vi "graphs B (SubVI).vi"(10 "Cluster":T1) -> ()   [LabVIEW 2015]
uses:
  Load and Save Controls_LV2009.llb/RWC_Actions.ctl
  <vilib>/Utility/error.llb/DialogType.ctl
panel:
  out "1":dynamicdata(graph) caption="U, uV"
  out "2":dynamicdata(graph) caption="U, uV"
  out "3":dynamicdata(graph) caption="U, uV"
  out "4":dynamicdata(graph) caption="U, uV"
  out "5":dynamicdata(graph) caption="U, uV"
  out "6":dynamicdata(graph) caption="U, uV"
  out "7":dynamicdata(graph) caption="U, uV"
  out "8":dynamicdata(graph) caption="U, uV"
  in  "clrear graphs":bool
  in  "4 sc":bool=TRUE
  in  "5 sc":bool=TRUE
  in  "7 sc":bool=TRUE
  in  "1 sc":bool=TRUE
  in  "2 sc":bool=TRUE
  in  "3 sc":bool=TRUE
  in  "6 sc":bool=TRUE
  in  "8 sc":bool=TRUE
  in  "4":bool=TRUE
  in  "5":bool
  in  "7":bool
  in  "1":bool=TRUE
  in  "2":bool=TRUE
  in  "3":bool=TRUE
  in  "6":bool
  in  "8":bool
  in  "dec time":bool
  in  "inc time":bool
  in  "Добавить время":dbl(ring)=300.0 items=["1 мин."=60.0, "5 мин."=300.0, "20 мин."=1200.0]
  out "мин.":string="1"
  out "часы":string="0"
  # "№ канала"
  # ":"
  # "Вкл."
  # "Автошкала"
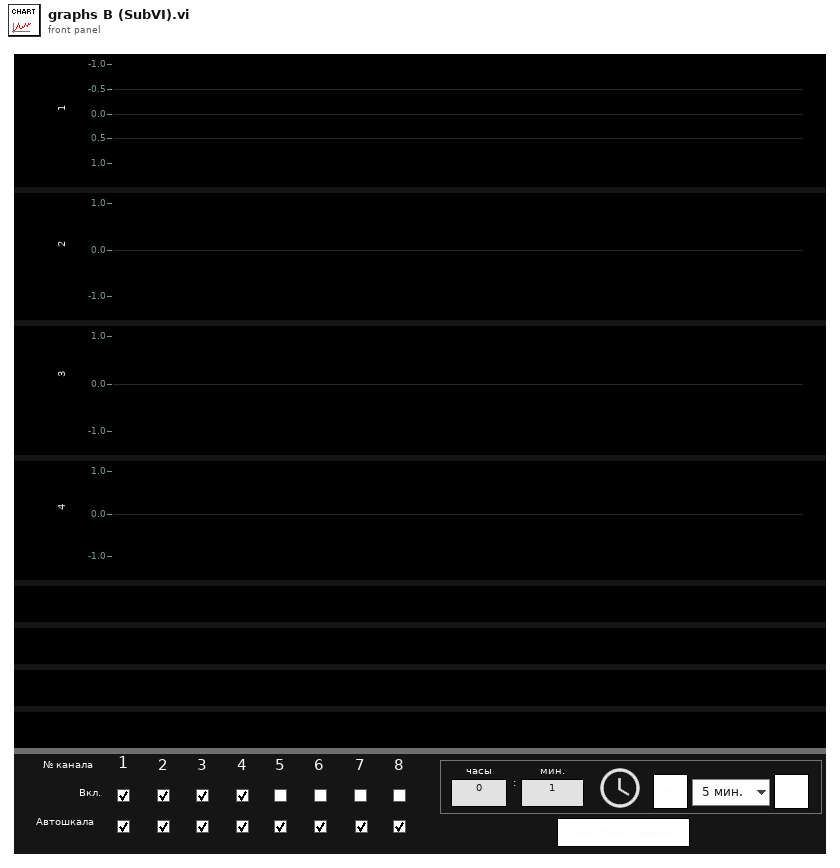
[diagram p1: front panel]
types:
  T1 = cluster{"1":dbl, "2":dbl, "3":dbl, "4":dbl, "5":dbl, "6":dbl, "7":dbl, "8":dbl}
  T2 = typedef "LVDateTimeRec.ctl" = cluster{"fractional second":dbl, "second":i32, "minute":i32, "hour":i32, "day of month":i32, "month":i32, "year":i32, "day of week":i32, "day of year":i32, "DST":i32}
  T3 = typedef "RWC_Actions.ctl" = enum16{"Read", "Write", "Read and Create"}
  T4 = typedef "DialogType.ctl" = u16
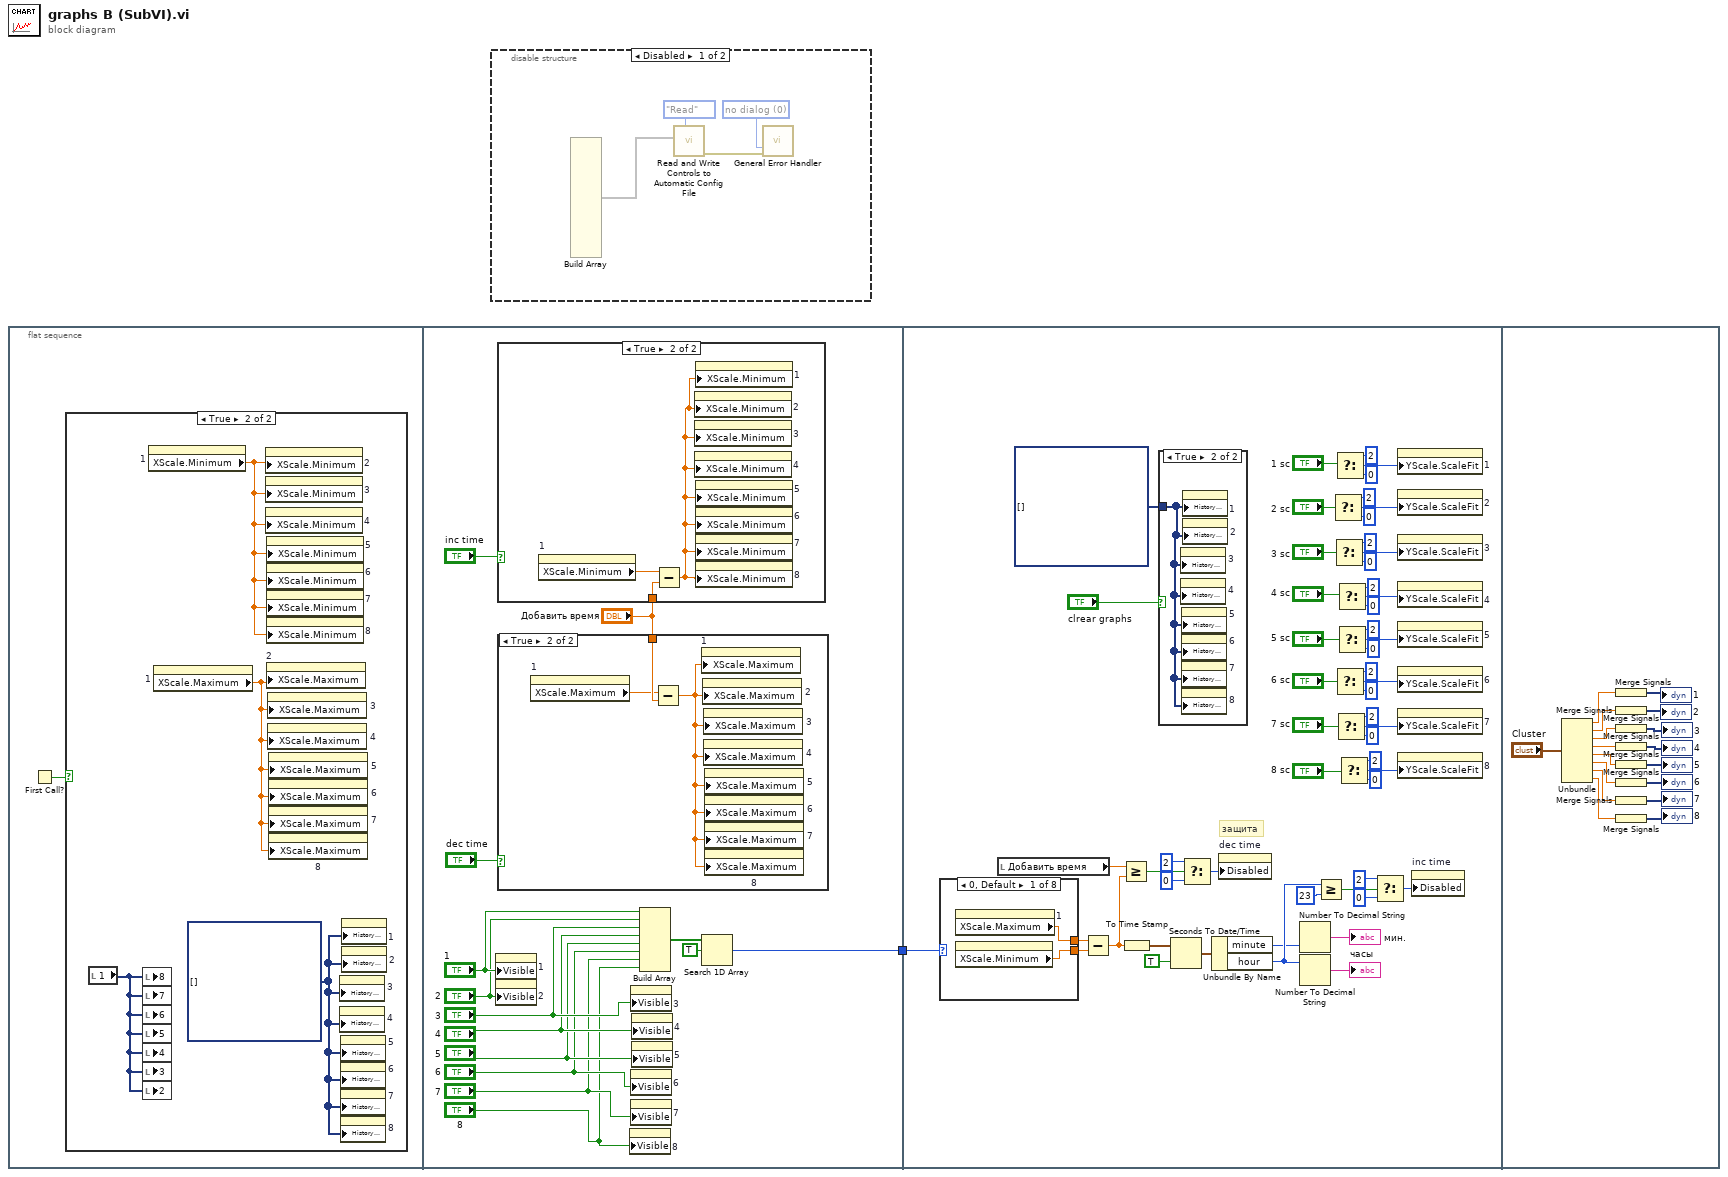
[diagram p0: block diagram]
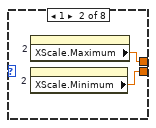
[diagram p7: hidden frame]
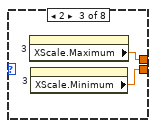
[diagram p8: hidden frame]
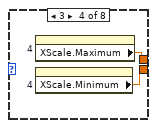
[diagram p9: hidden frame]
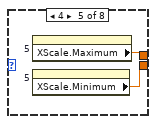
[diagram p10: hidden frame]
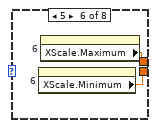
[diagram p11: hidden frame]
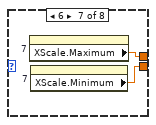
[diagram p12: hidden frame]
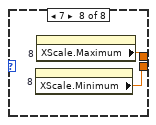
[diagram p13: hidden frame]
diagram:
  n1 = flat-sequence {
    tunnel: [w7] -> w1
    tunnel: w1 -> [w61]
    frame #0 {
      n2 = First Call?() -> (First Call?: T/F=w2:bool)
      n3 = case shown="True" w2 {
        frame False {
        }
        frame True {
          w6 = dynamicdata[] [] ("History Data")
          n4 = local read "1"() -> (w5:dynamicdata)
          n5 = local write "8"(w5) -> ()
          n6 = local write "7"(w5) -> ()
          n7 = local write "6"(w5) -> ()
          n8 = local write "5"(w5) -> ()
          n9 = local write "4"(w5) -> ()
          n10 = local write "3"(w5) -> ()
          n11 = local write "2"(w5) -> ()
          n12 = property on="1" class="WFChart (strict)"() -> ("XScale.Minimum"=w4:dbl)  [unwired: 2 in, 2 out]
          n13 = property on="1" class="WFChart (strict)"() -> ("XScale.Maximum"=w3:dbl)  [unwired: 2 in, 2 out]
          n14 = property on="2" class="WFChart (strict)"("XScale.Minimum"=w4) -> ()  [unwired: 2 in, 2 out]
          n15 = property on="3" class="WFChart (strict)"("XScale.Minimum"=w4) -> ()  [unwired: 2 in, 2 out]
          n16 = property on="4" class="WFChart (strict)"("XScale.Minimum"=w4) -> ()  [unwired: 2 in, 2 out]
          n17 = property on="5" class="WFChart (strict)"("XScale.Minimum"=w4) -> ()  [unwired: 2 in, 2 out]
          n18 = property on="6" class="WFChart (strict)"("XScale.Minimum"=w4) -> ()  [unwired: 2 in, 2 out]
          n19 = property on="7" class="WFChart (strict)"("XScale.Minimum"=w4) -> ()  [unwired: 2 in, 2 out]
          n20 = property on="8" class="WFChart (strict)"("XScale.Minimum"=w4) -> ()  [unwired: 2 in, 2 out]
          n21 = property on="2" class="WFChart (strict)"("XScale.Maximum"=w3) -> ()  [unwired: 2 in, 2 out]
          n22 = property on="3" class="WFChart (strict)"("XScale.Maximum"=w3) -> ()  [unwired: 2 in, 2 out]
          n23 = property on="4" class="WFChart (strict)"("XScale.Maximum"=w3) -> ()  [unwired: 2 in, 2 out]
          n24 = property on="5" class="WFChart (strict)"("XScale.Maximum"=w3) -> ()  [unwired: 2 in, 2 out]
          n25 = property on="6" class="WFChart (strict)"("XScale.Maximum"=w3) -> ()  [unwired: 2 in, 2 out]
          n26 = property on="7" class="WFChart (strict)"("XScale.Maximum"=w3) -> ()  [unwired: 2 in, 2 out]
          n27 = property on="8" class="WFChart (strict)"("XScale.Maximum"=w3) -> ()  [unwired: 2 in, 2 out]
          n28 = property on="3" class="WFChart (strict)"("History Data"=w6) -> ()  [unwired: 2 in, 2 out]
          n29 = property on="4" class="WFChart (strict)"("History Data"=w6) -> ()  [unwired: 2 in, 2 out]
          n30 = property on="5" class="WFChart (strict)"("History Data"=w6) -> ()  [unwired: 2 in, 2 out]
          n31 = property on="6" class="WFChart (strict)"("History Data"=w6) -> ()  [unwired: 2 in, 2 out]
          n32 = property on="7" class="WFChart (strict)"("History Data"=w6) -> ()  [unwired: 2 in, 2 out]
          n33 = property on="8" class="WFChart (strict)"("History Data"=w6) -> ()  [unwired: 2 in, 2 out]
          n34 = property on="1" class="WFChart (strict)"("History Data"=w6) -> ()  [unwired: 2 in, 2 out]
          n35 = property on="2" class="WFChart (strict)"("History Data"=w6) -> ()  [unwired: 2 in, 2 out]
        }
      }
    }
    frame #1 {
      n36 = property on="1" class="WFChart (strict)"("Visible"="1") -> ()  [unwired: 2 in, 2 out]
      n37 = property on="2" class="WFChart (strict)"("Visible"="2") -> ()  [unwired: 2 in, 2 out]
      n38 = case shown="True" "inc time" {
        tunnel: "Добавить время" -> [_ w26]
        frame False {
        }
        frame True {
          n39 = property on="1" class="WFChart (strict)"() -> ("XScale.Minimum"=w25:dbl)  [unwired: 2 in, 2 out]
          n40 = Subtract(x=w25, y=w26) -> (x-y=w24:dbl)
          n41 = property on="2" class="WFChart (strict)"("XScale.Minimum"=w24) -> ()  [unwired: 2 in, 2 out]
          n42 = property on="3" class="WFChart (strict)"("XScale.Minimum"=w24) -> ()  [unwired: 2 in, 2 out]
          n43 = property on="4" class="WFChart (strict)"("XScale.Minimum"=w24) -> ()  [unwired: 2 in, 2 out]
          n44 = property on="1" class="WFChart (strict)"("XScale.Minimum"=w24) -> ()  [unwired: 2 in, 2 out]
          n45 = property on="5" class="WFChart (strict)"("XScale.Minimum"=w24) -> ()  [unwired: 2 in, 2 out]
          n46 = property on="6" class="WFChart (strict)"("XScale.Minimum"=w24) -> ()  [unwired: 2 in, 2 out]
          n47 = property on="7" class="WFChart (strict)"("XScale.Minimum"=w24) -> ()  [unwired: 2 in, 2 out]
          n48 = property on="8" class="WFChart (strict)"("XScale.Minimum"=w24) -> ()  [unwired: 2 in, 2 out]
        }
      }
      n49 = case shown="True" "dec time" {
        tunnel: "Добавить время" -> [_ w23]
        frame False {
        }
        frame True {
          n50 = property on="1" class="WFChart (strict)"() -> ("XScale.Maximum"=w22:dbl)  [unwired: 2 in, 2 out]
          n51 = Subtract(x=w22, y=w23) -> (x-y=w21:dbl)
          n52 = property on="1" class="WFChart (strict)"("XScale.Maximum"=w21) -> ()  [unwired: 2 in, 2 out]
          n53 = property on="2" class="WFChart (strict)"("XScale.Maximum"=w21) -> ()  [unwired: 2 in, 2 out]
          n54 = property on="3" class="WFChart (strict)"("XScale.Maximum"=w21) -> ()  [unwired: 2 in, 2 out]
          n55 = property on="4" class="WFChart (strict)"("XScale.Maximum"=w21) -> ()  [unwired: 2 in, 2 out]
          n56 = property on="5" class="WFChart (strict)"("XScale.Maximum"=w21) -> ()  [unwired: 2 in, 2 out]
          n57 = property on="6" class="WFChart (strict)"("XScale.Maximum"=w21) -> ()  [unwired: 2 in, 2 out]
          n58 = property on="7" class="WFChart (strict)"("XScale.Maximum"=w21) -> ()  [unwired: 2 in, 2 out]
          n59 = property on="8" class="WFChart (strict)"("XScale.Maximum"=w21) -> ()  [unwired: 2 in, 2 out]
        }
      }
      n60 = property on="8" class="WFChart (strict)"("Visible"="8") -> ()  [unwired: 2 in, 2 out]
      n61 = property on="3" class="WFChart (strict)"("Visible"="3") -> ()  [unwired: 2 in, 2 out]
      n62 = property on="6" class="WFChart (strict)"("Visible"="6") -> ()  [unwired: 2 in, 2 out]
      n63 = property on="7" class="WFChart (strict)"("Visible"="7") -> ()  [unwired: 2 in, 2 out]
      n64 = property on="4" class="WFChart (strict)"("Visible"="4") -> ()  [unwired: 2 in, 2 out]
      n65 = property on="5" class="WFChart (strict)"("Visible"="5") -> ()  [unwired: 2 in, 2 out]
      n66 = Build Array("1", "2", "3", "4", "5", "6", "7", "8") -> (w9:bool[])
      n67 = Search 1D Array(1D array=w9, element=TRUE) -> (index of element=w7:i32)  [unwired: 1 in]
    }
    frame #2 {
      # "защита"
      n68 = case shown="0, Default" w61 {
        tunnel: [w84 w86 w88 w90 w92 w94 w96 w98] -> w63
        tunnel: [w83 w85 w87 w89 w91 w93 w95 w97] -> w62
        frame 0, Default {
          n69 = property on="1" class="WFChart (strict)"() -> ("XScale.Maximum"=w84:dbl)  [unwired: 2 in, 2 out]
          n70 = property on="1" class="WFChart (strict)"() -> ("XScale.Minimum"=w83:dbl)  [unwired: 2 in, 2 out]
        }
        frame 1 {
          n71 = property on="2" class="WFChart (strict)"() -> ("XScale.Maximum"=w86:dbl)  [unwired: 2 in, 2 out]
          n72 = property on="2" class="WFChart (strict)"() -> ("XScale.Minimum"=w85:dbl)  [unwired: 2 in, 2 out]
        }
        frame 2 {
          n73 = property on="3" class="WFChart (strict)"() -> ("XScale.Maximum"=w88:dbl)  [unwired: 2 in, 2 out]
          n74 = property on="3" class="WFChart (strict)"() -> ("XScale.Minimum"=w87:dbl)  [unwired: 2 in, 2 out]
        }
        frame 3 {
          n75 = property on="4" class="WFChart (strict)"() -> ("XScale.Maximum"=w90:dbl)  [unwired: 2 in, 2 out]
          n76 = property on="4" class="WFChart (strict)"() -> ("XScale.Minimum"=w89:dbl)  [unwired: 2 in, 2 out]
        }
        frame 4 {
          n77 = property on="5" class="WFChart (strict)"() -> ("XScale.Maximum"=w92:dbl)  [unwired: 2 in, 2 out]
          n78 = property on="5" class="WFChart (strict)"() -> ("XScale.Minimum"=w91:dbl)  [unwired: 2 in, 2 out]
        }
        frame 5 {
          n79 = property on="6" class="WFChart (strict)"() -> ("XScale.Minimum"=w93:dbl)  [unwired: 2 in, 2 out]
          n80 = property on="6" class="WFChart (strict)"() -> ("XScale.Maximum"=w94:dbl)  [unwired: 2 in, 2 out]
        }
        frame 6 {
          n81 = property on="7" class="WFChart (strict)"() -> ("XScale.Maximum"=w96:dbl)  [unwired: 2 in, 2 out]
          n82 = property on="7" class="WFChart (strict)"() -> ("XScale.Minimum"=w95:dbl)  [unwired: 2 in, 2 out]
        }
        frame 7 {
          n83 = property on="8" class="WFChart (strict)"() -> ("XScale.Minimum"=w97:dbl)  [unwired: 2 in, 2 out]
          n84 = property on="8" class="WFChart (strict)"() -> ("XScale.Maximum"=w98:dbl)  [unwired: 2 in, 2 out]
        }
      }
      n85 = local read "Добавить время"() -> (w64:dbl)
      n86 = Subtract(x=w63, y=w62) -> (x-y=w71:dbl)
      n87 = Greater Or Equal?(x=w64, y=w71) -> (x >= y?=w77:bool)
      n88 = To Time Stamp(1:w71) -> (0:w66:timestamp)
      n89 = case shown="True" "clrear graphs" {
        tunnel: dynamicdata[] [] ("History Data") -> [_ w82]
        frame False {
        }
        frame True {
          n90 = property on="3" class="WFChart (strict)"("History Data"=w82) -> ()  [unwired: 2 in, 2 out]
          n91 = property on="4" class="WFChart (strict)"("History Data"=w82) -> ()  [unwired: 2 in, 2 out]
          n92 = property on="5" class="WFChart (strict)"("History Data"=w82) -> ()  [unwired: 2 in, 2 out]
          n93 = property on="6" class="WFChart (strict)"("History Data"=w82) -> ()  [unwired: 2 in, 2 out]
          n94 = property on="7" class="WFChart (strict)"("History Data"=w82) -> ()  [unwired: 2 in, 2 out]
          n95 = property on="8" class="WFChart (strict)"("History Data"=w82) -> ()  [unwired: 2 in, 2 out]
          n96 = property on="1" class="WFChart (strict)"("History Data"=w82) -> ()  [unwired: 2 in, 2 out]
          n97 = property on="2" class="WFChart (strict)"("History Data"=w82) -> ()  [unwired: 2 in, 2 out]
        }
      }
      n98 = Seconds To Date/Time(time stamp (now)=w66, to UTC (F)=TRUE) -> (date time rec=w67:T2)
      n99 = Select(t=u8 2 ("Disabled"), s=w77, f=u8 0 ("Disabled")) -> (s? t:f=w74:u8)
      n100 = Unbundle By Name(w67) -> ("minute"=w68:i32, "hour"=w72:i32)
      n101 = property on="dec time" class="Bool"("Disabled"=w74) -> ()  [unwired: 2 in, 2 out]
      n102 = Number To Decimal String(number=w68) -> (decimal integer string=→"мин.":string)  [unwired: 1 out]
      n103 = Number To Decimal String(number=w72) -> (decimal integer string=→"часы":string)  [unwired: 1 out]
      n104 = Greater Or Equal?(x=w72, y=23) -> (x >= y?=w81:bool)
      n105 = Select(t=u8 2 ("Y Scale.Scale Fit"), s="2 sc", f=u8 0 ("Y Scale.Scale Fit")) -> (s? t:f=w53:u8)
      n106 = Select(t=u8 2 ("Y Scale.Scale Fit"), s="3 sc", f=u8 0 ("Y Scale.Scale Fit")) -> (s? t:f=w49:u8)
      n107 = Select(t=u8 2 ("Y Scale.Scale Fit"), s="1 sc", f=u8 0 ("Y Scale.Scale Fit")) -> (s? t:f=w60:u8)
      n108 = Select(t=u8 2 ("Y Scale.Scale Fit"), s="6 sc", f=u8 0 ("Y Scale.Scale Fit")) -> (s? t:f=w33:u8)
      n109 = Select(t=u8 2 ("Y Scale.Scale Fit"), s="7 sc", f=u8 0 ("Y Scale.Scale Fit")) -> (s? t:f=w35:u8)
      n110 = Select(t=u8 2 ("Y Scale.Scale Fit"), s="4 sc", f=u8 0 ("Y Scale.Scale Fit")) -> (s? t:f=w45:u8)
      n111 = Select(t=u8 2 ("Y Scale.Scale Fit"), s="5 sc", f=u8 0 ("Y Scale.Scale Fit")) -> (s? t:f=w34:u8)
      n112 = Select(t=u8 2 ("Y Scale.Scale Fit"), s="8 sc", f=u8 0 ("Y Scale.Scale Fit")) -> (s? t:f=w36:u8)
      n113 = Select(t=u8 2 ("Disabled"), s=w81, f=u8 0 ("Disabled")) -> (s? t:f=w78:u8)
      n114 = property on="1" class="WFChart (strict)"("YScale.ScaleFit"=w60) -> ()  [unwired: 2 in, 2 out]
      n115 = property on="2" class="WFChart (strict)"("YScale.ScaleFit"=w53) -> ()  [unwired: 2 in, 2 out]
      n116 = property on="3" class="WFChart (strict)"("YScale.ScaleFit"=w49) -> ()  [unwired: 2 in, 2 out]
      n117 = property on="4" class="WFChart (strict)"("YScale.ScaleFit"=w45) -> ()  [unwired: 2 in, 2 out]
      n118 = property on="5" class="WFChart (strict)"("YScale.ScaleFit"=w34) -> ()  [unwired: 2 in, 2 out]
      n119 = property on="6" class="WFChart (strict)"("YScale.ScaleFit"=w33) -> ()  [unwired: 2 in, 2 out]
      n120 = property on="7" class="WFChart (strict)"("YScale.ScaleFit"=w35) -> ()  [unwired: 2 in, 2 out]
      n121 = property on="8" class="WFChart (strict)"("YScale.ScaleFit"=w36) -> ()  [unwired: 2 in, 2 out]
      n122 = property on="inc time" class="Bool"("Disabled"=w78) -> ()  [unwired: 2 in, 2 out]
    }
    frame #3 {
      n123 = Unbundle("Cluster") -> ("1"=w108:dbl, "2"=w109:dbl, "3"=w110:dbl, "4"=w111:dbl, "5"=w112:dbl, "6"=w113:dbl, "7"=w114:dbl, "8"=w115:dbl)
      n124 = Merge Signals(w108) -> (→"1":dynamicdata)
      n125 = Merge Signals(w109) -> (→"2":dynamicdata)
      n126 = Merge Signals(w110) -> (→"3":dynamicdata)
      n127 = Merge Signals(w111) -> (→"4":dynamicdata)
      n128 = Merge Signals(w112) -> (→"5":dynamicdata)
      n129 = Merge Signals(w113) -> (→"6":dynamicdata)
      n130 = Merge Signals(w114) -> (→"7":dynamicdata)
      n131 = Merge Signals(w115) -> (→"8":dynamicdata)
    }
  }
  n132 = disable-structure shown="Disabled" {
    frame Disabled {
      w117 = T4 0 items=["no dialog", "OK message", "continue or stop message", "OK message + warnings", "continue/stop + warnings"] ("type of dialog (OK msg:1)")
      n133 = Build Array() -> (w116:void[])  [unwired: 15 in]
      n134 = call "Read and Write Controls to Automatic Config File.vi"("Action"=RWC_Actions."Read", "Control References"=w116) -> ("error out"=w118:errorcluster)  [unwired: 9 in]
      n135 = call <vilib>:"General Error Handler.vi"("type of dialog (OK msg:1)"=w117, "error in (no error)"=w118) -> ()  [unwired: 1 in, 13 out]
    }
    frame Enabled {
    }
  }
